vi "Server Errors.vi"() -> ()   [LabVIEW 2017]
panel:
  out "invalid params":errorcluster={"status"=TRUE, "code"=-32602, "source"="Invalid params"}
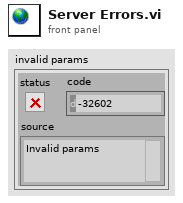
[diagram p1: front panel]
diagram:
